vi "纳清电导率_所有参数读取.vi"(8 "error in (no error)":errorcluster caption="错误输入（无错误）", 11 "MB session in":refnum<class "MB_Master.lvclass">) -> (0 "error out":errorcluster caption="错误输出", 2 "输出值":T1 {"波特率" items=["4800", "9600", "19200", "38400", "57600", "115200"]}, 3 "MB session out":refnum<class "MB_Master.lvclass">)   [LabVIEW 2016, in "斯坦道多参数.lvlib"]
uses:
  <vilib>/Plasmionique/MB Master/MB_Master/MB_Master.lvclass
  <vilib>/Plasmionique/MB Master/MB Master.lvlib
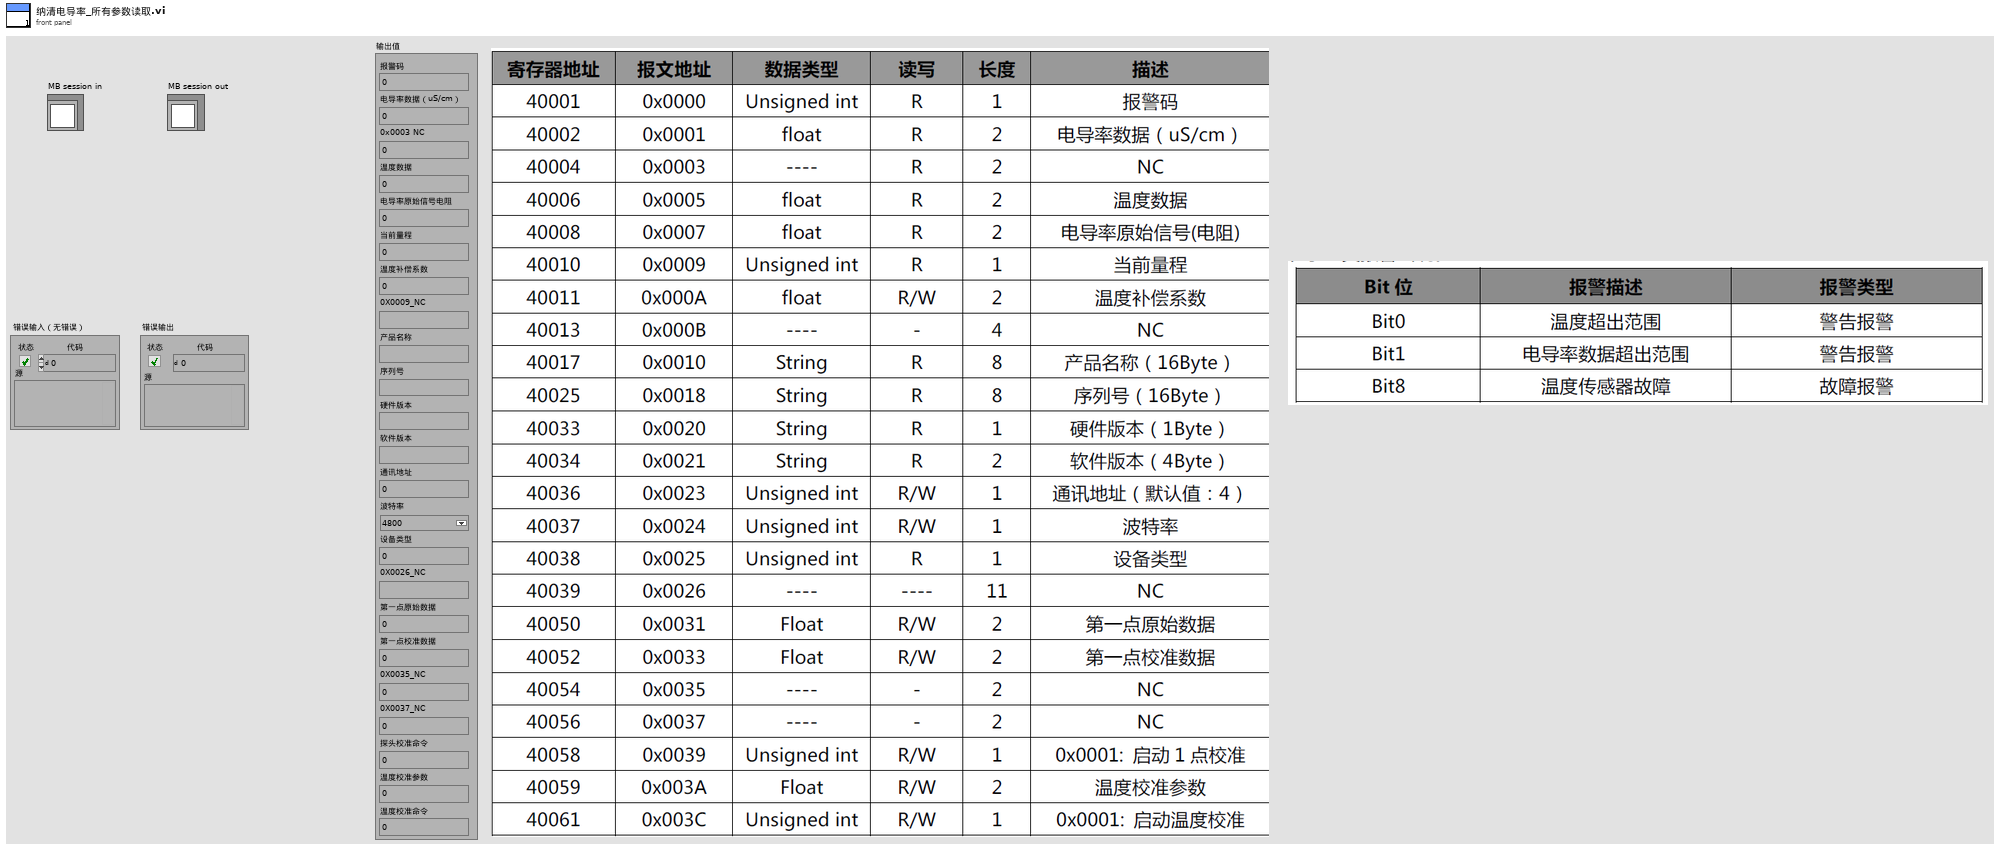
[diagram p1: front panel]
types:
  T1 = cluster{"报警码":u16, "电导率数据（uS/cm）":sgl, "0x0003 NC":sgl, "温度数据":sgl, "电导率原始信号电阻":sgl, "当前量程":u16, "温度补偿系数":sgl, "0X0009_NC":string, "产品名称":string, "序列号":string, "硬件版本":string, "软件版本":string, "通讯地址":u16, "波特率":u16, "设备类型":u16, "0X0026_NC":string, "第一点原始数据":sgl, "第一点校准数据":sgl, "0X0035_NC":sgl, "0X0037_NC":sgl, "探头校准命令":u16, "温度校准参数":sgl, "温度校准命令":u16}
  T2 = cluster{"pH":u32, "DO":u32, "Cond":u32, "Turb":u32, "叶绿素a":u32, "藻密度":u32, "ORP":u32, "COD":u32, "氯化物":u32, "氨氮":u32, "水中油":u32, "悬浮物":u32, "余氯":u32}
  T3 = cluster{u16, "mode":dbl, "数值":sgl, "数值":sgl, "数值":sgl, u16, "数值":sgl, "类型":string, "类型":string, "类型":string, "类型":string, "类型":string, u16, u16, u16, "类型":string, "数值":sgl, "数值":sgl, "数值":sgl, "数值":sgl, u16, "数值":sgl, u16}
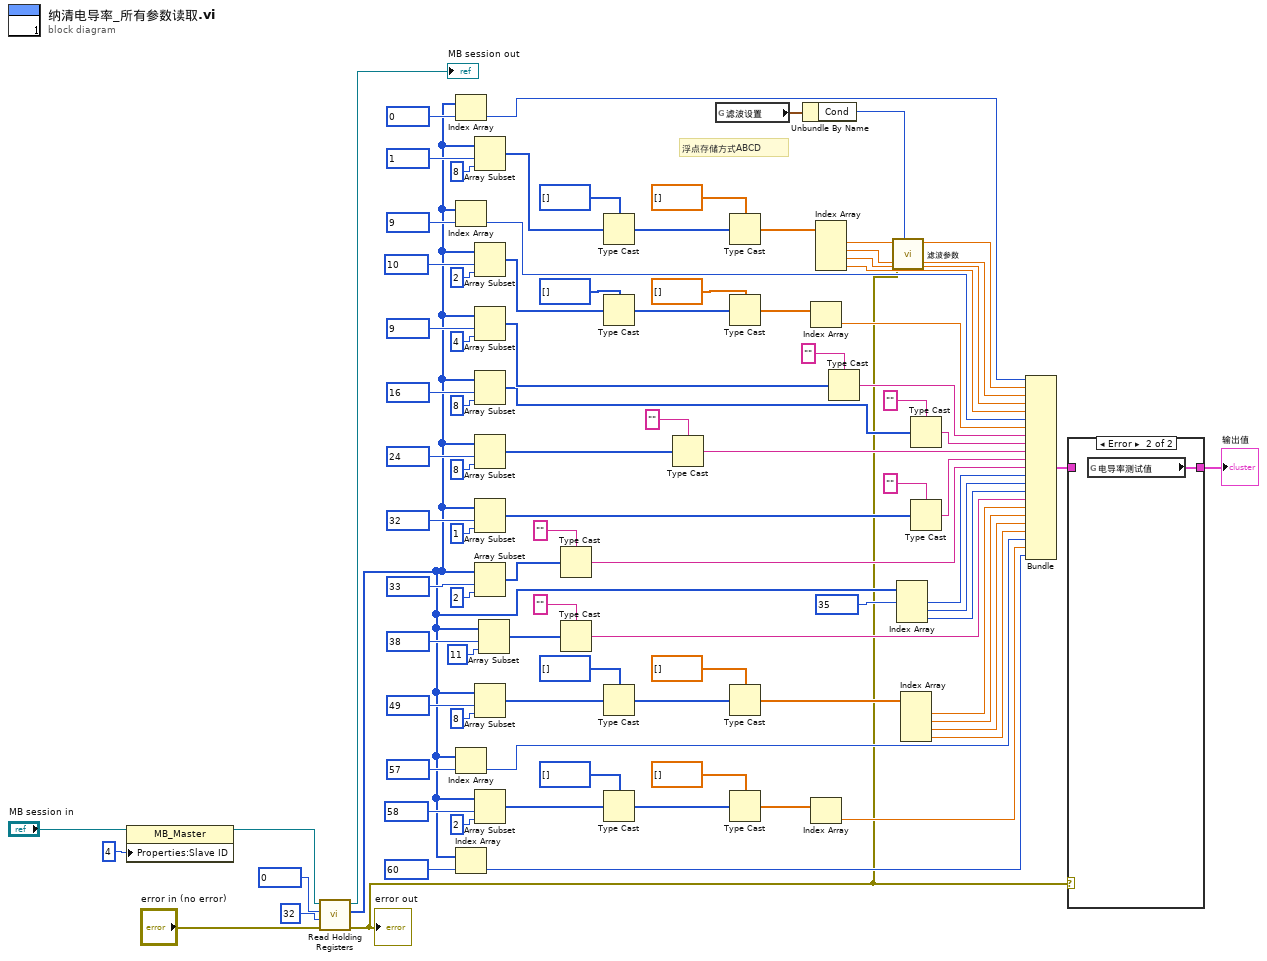
[diagram p0: block diagram]
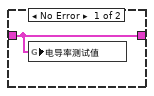
[diagram p2: hidden frame]
diagram:
  # "浮点存储方式ABCD"
  n1 = property class="MB_Master"(reference="MB session in", "Properties:Slave ID"=u8 4 ("Slave ID")) -> (reference out=w84:refnum<class "MB_Master.lvclass">)  [unwired: 1 in, 1 out]
  n2 = call <vilib>:"Read Holding Registers.vi"("error in (no error)"="error in (no error)", "quantity"=u16 32, "starting address"=u16 0, "MB session in"=w84) -> ("error out"=w1:errorcluster, "Registers"=w8:u16[], "MB session out"=→"MB session out":refnum<class "MB_Master.lvclass">)  [unwired: 5 in]
  "error out" <- w1
  n3 = Index Array(array=w8, index=u16 0 ("starting address")) -> (element=w92:u16)
  n4 = Index Array(array=w8, index=u16 9 ("starting address")) -> (element=w7:u16)
  n5 = Index Array(array=w8, index=u16 57 ("starting address")) -> (element=w30:u16)
  n6 = Index Array(array=w8, index=u16 60 ("starting address")) -> (element=w27:u16)
  n7 = Array Subset(array=w8, index=u16 1 ("starting address"), length=8 ("长度")) -> (w88:u16[])
  n8 = Array Subset(array=w8, index=u16 10 ("starting address"), length=2 ("长度")) -> (w11:u16[])
  n9 = Array Subset(array=w8, index=u16 9 ("starting address"), length=4 ("长度")) -> (w78:u16[])
  n10 = Array Subset(array=w8, index=u16 16 ("starting address"), length=8 ("长度")) -> (w74:u16[])
  n11 = Array Subset(array=w8, index=u16 24 ("starting address"), length=8 ("长度")) -> (w68:u16[])
  n12 = Array Subset(array=w8, index=u16 32 ("starting address"), length=1 ("长度")) -> (w64:u16[])
  n13 = Array Subset(array=w8, index=u16 33 ("starting address"), length=2 ("长度")) -> (w58:u16[])
  n14 = Array Subset(array=w8, index=u16 49 ("starting address"), length=8 ("长度")) -> (w45:u16[])
  n15 = Array Subset(array=w8, index=u16 58 ("starting address"), length=2 ("长度")) -> (w33:u16[])
  n16 = Array Subset(array=w8, index=u16 38 ("starting address"), length=11 ("长度")) -> (w48:u16[])
  n17 = Type Cast(type="" ("类型"), x=w58) -> (*(type *) &x=w56:string)
  n18 = Type Cast(type="" ("类型"), x=w48) -> (*(type *) &x=w47:string)
  n19 = Type Cast(type=u32[] [] ("数组 2"), x=w88) -> (*(type *) &x=w26:u32[])
  n20 = Type Cast(type=u32[] [] ("数组 2"), x=w11) -> (*(type *) &x=w15:u32[])
  n21 = Type Cast(type=u32[] [] ("数组 2"), x=w45) -> (*(type *) &x=w43:u32[])
  n22 = Type Cast(type=u32[] [] ("数组 2"), x=w33) -> (*(type *) &x=w35:u32[])
  n23 = Type Cast(type="" ("类型"), x=w68) -> (*(type *) &x=w66:string)
  n24 = global read "断电保存变量.vi" "滤波设置"() -> (w4:T2)
  n25 = Type Cast(type=sgl[] [] ("数组 2"), x=w26) -> (*(type *) &x=w87:sgl[])
  n26 = Type Cast(type=sgl[] [] ("数组 2"), x=w15) -> (*(type *) &x=w14:sgl[])
  n27 = Type Cast(type=sgl[] [] ("数组 2"), x=w43) -> (*(type *) &x=w40:sgl[])
  n28 = Type Cast(type=sgl[] [] ("数组 2"), x=w35) -> (*(type *) &x=w38:sgl[])
  n29 = Unbundle By Name(w4) -> ("Cond"=w3:u32)
  n30 = Index Array(array=w14) -> (element=w10:sgl)  [unwired: 1 in]
  n31 = Index Array(array=w38) -> (element=w29:sgl)  [unwired: 1 in]
  n32 = Index Array(array=w87) -> (element #1=w6:sgl, element #2=w82:sgl, element #3=w23:sgl, element #4=w22:sgl)  [unwired: 4 in]
  n33 = Type Cast(type="" ("类型"), x=w78) -> (*(type *) &x=w76:string)
  n34 = call "滤波参数.vi"("滤波次数"=w3, "error in (no error)"=w1, "x"=w6) -> ("mode"=w5:dbl)  [unwired: 7 in, 1 out]
  n35 = Index Array(array=w8, index #1=u16 35 ("starting address")) -> (element #1=w54:u16, element #2=w53:u16, element #3=w52:u16)  [unwired: 2 in]
  n36 = Index Array(array=w40) -> (element #1=w39:sgl, element #2=w21:sgl, element #3=w20:sgl, element #4=w19:sgl)  [unwired: 4 in]
  n37 = Type Cast(type="" ("类型"), x=w74) -> (*(type *) &x=w71:string)
  n38 = Type Cast(type="" ("类型"), x=w64) -> (*(type *) &x=w61:string)
  n39 = Bundle(w92, "mode"=w5, "数值"=w82, "数值"=w23, "数值"=w22, w7, "数值"=w10, "类型"=w76, "类型"=w71, "类型"=w66, "类型"=w61, "类型"=w56, w54, w53, w52, "类型"=w47, "数值"=w39, "数值"=w21, "数值"=w20, "数值"=w19, w30, "数值"=w29, w27) -> (w18:T3)  [unwired: 1 in]
  n40 = case shown="Error" w1 {
    tunnel: w18 -> [w95 _]
    tunnel: [w95 w96] -> w2
    frame No Error {
      n41 = global write "纳清过程全局变量.vi" "电导率测试值"(w95) -> ()
    }
    frame Error {
      n42 = global read "纳清过程全局变量.vi" "电导率测试值"() -> (w96:T1)
    }
  }
  "输出值" <- w2
